vi "4461 - Create AO waveforms.vi"(8 "error in (no error)":errorcluster, 10 "reset phase":bool, 11 "Lockin.DAQ":refnum<class "Lockin.DAQ.lvclass">) -> (0 "error out":errorcluster, 2 "AO Array":waveform(dbl)[](array[waveform]), 3 "Lockin.DAQ":refnum<class "Lockin.DAQ.lvclass">)   [LabVIEW 2016, in "Lockin.DAQ.lvclass"]
uses:
  Lockin.DAQ.lvclass
  Typedefs/AO-cluster.ctl
  Instrument.Lockinl.UI/Typedefs/AO Channel--Cluster.ctl
  Typedefs/Function-enum.ctl
  Lockin.DAQ.lvclass/Lockin.DAQ.ctl
  <vilib>/measure/NI_MABase.lvlib
  Typedefs/Sampling.ctl
  Instrument.Lockinl.UI/Instrument.Lockin.UI.lvclass
panel:
  in  "Channels: AO":T1 {"Phase" format="%.3g"; "Frequency" min=0.0001 max=10000.0 format="%.3g"; "Offset" format="%.3p"; "Amplitude" min=0.0 max=10.0 format="%.3p"}
  in  "Update Graph?":bool
  out "Waveform Chart":dbl[][](graph)
  out "Waveform Graph":waveform(dbl)[](graph)
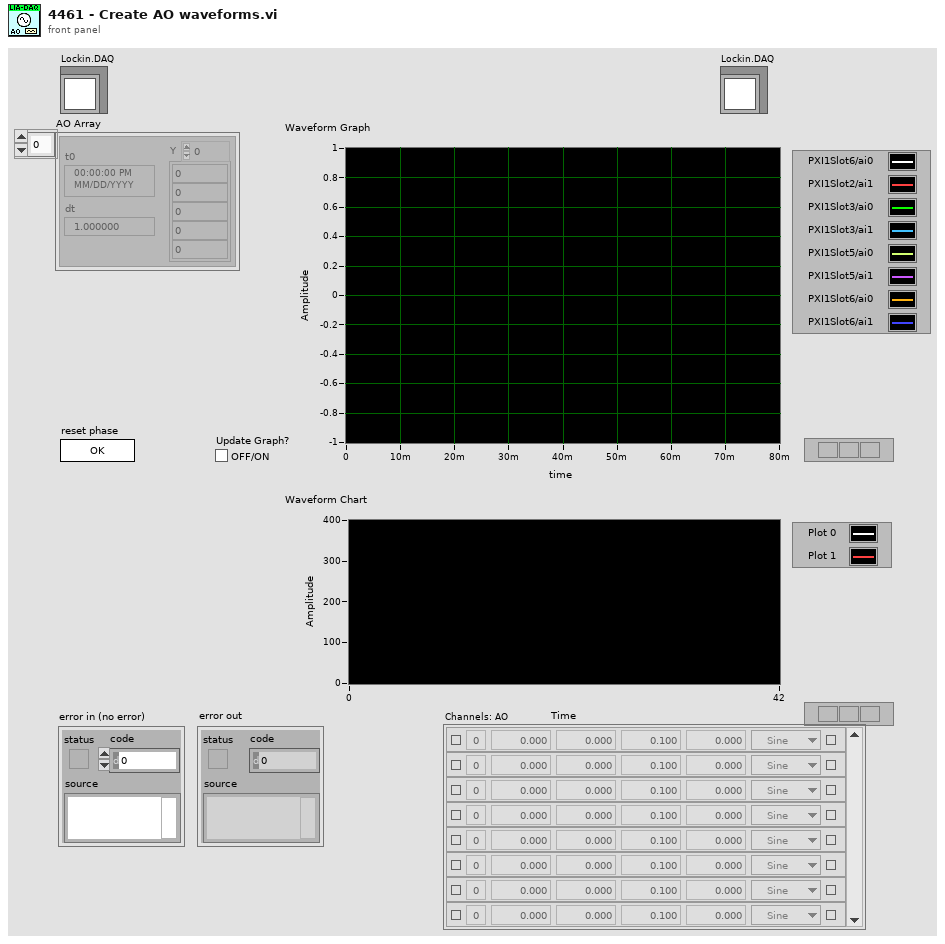
[diagram p1: front panel]
types:
  T1 = typedef "Lockin.DAQ.lvclass/AO-cluster.ctl" = T2[]
  T2 = typedef "Instrument.Lockin.UI.lvclass/AO Channel--Cluster.ctl" = cluster{"Enable?":bool, "Channel":i32, "Amplitude":dbl, "Offset":dbl, "Frequency":dbl, "Phase":dbl, "Function":T3, "Sweeping?":bool}
  T3 = typedef "Lockin.DAQ.lvclass/Function-enum.ctl" = enum16{"Sine", "Triangle", "Square"}
  T4 = typedef "Lockin.DAQ.lvclass/Sampling.ctl" = cluster{"Fs":dbl, "#s":i32}
  T5 = enum16{"Sine Wave", "Triangle Wave", "Square Wave", "Sawtooth Wave"}
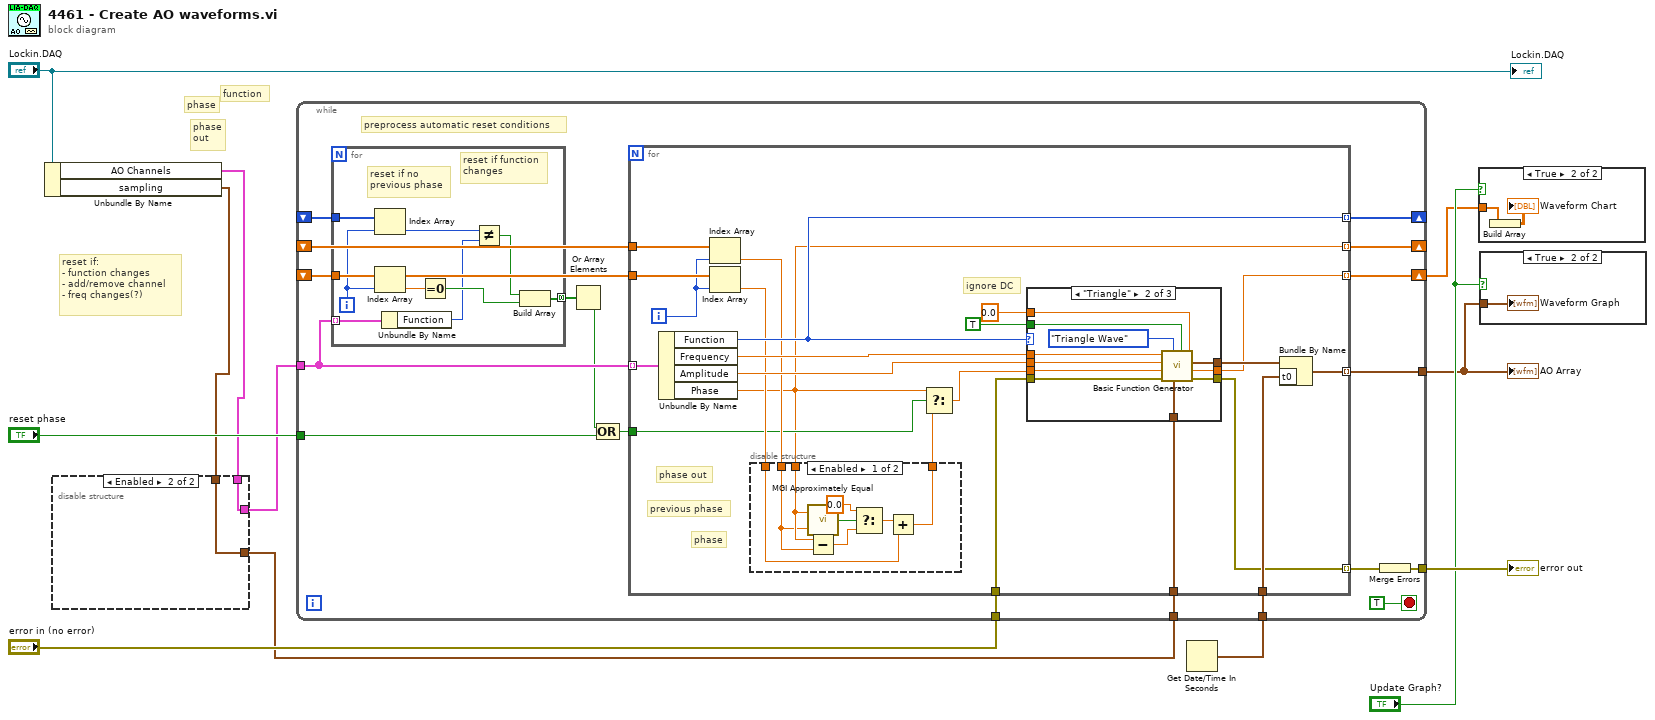
[diagram p0: block diagram]
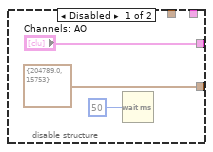
[diagram p2: hidden frame]
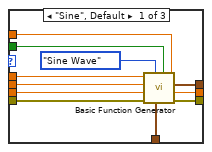
[diagram p4: hidden frame]
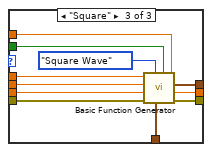
[diagram p5: hidden frame]
diagram:
  # "phase"
  # "function"
  # "phase\nout"
  # "reset if:\n- function changes\n- add/remove channel\n- freq changes(?)"
  n1 = Unbundle By Name("Lockin.DAQ") -> ("AO Channels"=w2:T1, "sampling"=w1:T4)
  n2 = disable-structure shown="Enabled" {
    disable-tunnel: [T4 {"Fs"=204789.0, "#s"=15753} ("Configuration.DAQ.sampling") w16] -> w4
    disable-tunnel: ["Channels: AO" w17] -> w3
    disable-tunnel: w2 -> [_ w17]
    disable-tunnel: w1 -> [_ w16]
    frame Disabled {
      n3 = Wait (ms)(milliseconds to wait=u32 50) -> ()  [unwired: 1 out]
    }
    frame Enabled {
    }
  }
  n4 = Get Date/Time In Seconds() -> (seconds since 1Jan1904=w11:timestamp)
  n5 = while {
    tunnel: w4 -> [w35]
    tunnel: [w34] -> w6
    shift-right: [w32] -> w5
    shift-left: _ -> [w20]
    tunnel: w11 -> [w31]
    tunnel: "reset phase" -> [w24]
    tunnel: "error in (no error)" -> [w30]
    tunnel: [w28] -> w10
    tunnel: w3 -> [w27]
    shift-right: [w22] -> _
    shift-left: _ -> [w21]
    shift-right: [w19] -> _
    shift-left: _ -> [w18]
    stop <- TRUE stop-if-true
    # "preprocess automatic reset conditions"
    n6 = for {
      tunnel: w27 -> [w37] mode=indexing
      tunnel: w20 -> [w44]
      tunnel: w21 -> [w43]
      tunnel: [w38] -> w26 mode=concatenating
      i -> [w45]
      # "reset if function\nchanges"
      # "reset if no\nprevious phase"
      n7 = Index Array(array=w43, index=w45) -> (element=w41:T3)
      n8 = Index Array(array=w44, index=w45) -> (element=w42:dbl)
      n9 = Unbundle By Name(w37) -> ("Function"=w36:T3)
      n10 = Equal To 0?(x=w42) -> (x = 0?=w39:bool)
      n11 = Not Equal?(x=w41, y=w36) -> (x != y?=w40:bool)
      n12 = Build Array(w40, w39) -> (w38:bool[])
    }
    n13 = Or Array Elements(Boolean array=w26) -> (logical OR=w25:bool)
    n14 = Compound Arithmetic op=OR(w25, w24) -> (w23:bool)
    n15 = for {
      tunnel: [w64] -> w34 mode=indexing
      tunnel: w35 -> [w61]
      tunnel: [w62] -> w32 mode=indexing
      tunnel: w31 -> [w66]
      tunnel: w30 -> [w59]
      tunnel: [w63] -> w29 mode=indexing
      tunnel: w27 -> [w58] mode=indexing
      tunnel: w23 -> [w47]
      tunnel: [w55] -> w22 mode=indexing
      tunnel: w20 -> [w54]
      tunnel: [w46] -> w19 mode=indexing
      tunnel: w18 -> [w50]
      i -> [w53]
      # "previous phase"
      # "phase"
      # "phase out"
      # "ignore DC"
      n16 = Unbundle By Name(w58) -> ("Function"=w55:T3, "Frequency"=w56:dbl, "Amplitude"=w57:dbl, "Phase"=w46:dbl)
      n17 = Index Array(array=w50, index=w53) -> (element=w51:dbl)
      n18 = Index Array(array=w54, index=w53) -> (element=w52:dbl)
      n19 = disable-structure shown="Enabled" {
        disable-tunnel: w46 -> [w74 _]
        disable-tunnel: w51 -> [w73 _]
        disable-tunnel: w52 -> [w68 w76]
        disable-tunnel: [w71 w76] -> w49
        frame Enabled {
          n20 = call <userlib>:"MGI Approximately Equal.vi"("Numeric 2"=w73, "Numeric 1"=w74) -> ("approx = ?"=w72:bool)
          n21 = Subtract(x=w74, y=w73) -> (x-y=w70:dbl)
          n22 = Select(t=0.0, s=w72, f=w70) -> (s? t:f=w69:dbl)
          n23 = Add(x=w69, y=w68) -> (x+y=w71:dbl)
        }
        frame Disabled {
        }
      }
      n24 = Select(t=w46, s=w47, f=w49) -> (s? t:f=w48:dbl)
      n25 = case shown="\"Triangle\"" w55 {
        tunnel: w56 -> [w87 w98 w109]
        tunnel: 0.0 ("AO DC") -> [w86 w97 w108]
        tunnel: [w85 w96 w107] -> w67
        tunnel: TRUE ("reset signal") -> [w77 w88 w99]
        tunnel: w59 -> [w84 w95 w106]
        tunnel: [w83 w94 w105] -> w63
        tunnel: [w82 w93 w104] -> w62
        tunnel: w57 -> [w81 w92 w103]
        tunnel: w48 -> [w80 w91 w102]
        tunnel: w61 -> [w79 w90 w101]
        frame "Sine", Default {
          n26 = call <vilib>:"Basic Function Generator.vi"("offset"=w86, "reset signal"=w77, "sampling info"=w79, "signal type"=T5."Sine Wave", "error in (no error)"=w84, "phase"=w80, "amplitude"=w81, "frequency"=w87) -> ("error out"=w83:errorcluster, "phase out"=w82:dbl, "signal out"=w85:waveform(dbl))  [unwired: 1 in]
        }
        frame "Triangle" {
          n27 = call <vilib>:"Basic Function Generator.vi"("offset"=w97, "reset signal"=w88, "sampling info"=w90, "signal type"=T5."Triangle Wave", "error in (no error)"=w95, "phase"=w91, "amplitude"=w92, "frequency"=w98) -> ("error out"=w94:errorcluster, "phase out"=w93:dbl, "signal out"=w96:waveform(dbl))  [unwired: 1 in]
        }
        frame "Square" {
          n28 = call <vilib>:"Basic Function Generator.vi"("offset"=w108, "reset signal"=w99, "sampling info"=w101, "signal type"=T5."Square Wave", "error in (no error)"=w106, "phase"=w102, "amplitude"=w103, "frequency"=w109) -> ("error out"=w105:errorcluster, "phase out"=w104:dbl, "signal out"=w107:waveform(dbl))  [unwired: 1 in]
        }
      }
      n29 = Bundle By Name(cluster=w67, "t0"=w66) -> (w64:waveform(dbl))
    }
    n30 = Merge Errors(w29) -> (w28:errorcluster)
  }
  "AO Array" <- w6
  "error out" <- w10
  n31 = case shown="True" "Update Graph?" {
    tunnel: w5 -> [_ w111]
    frame False {
    }
    frame True {
      n32 = Build Array(w111) -> (→"Waveform Chart":dbl[][])
    }
  }
  n33 = case shown="True" "Update Graph?" {
    tunnel: w6 -> [_ w112]
    frame False {
    }
    frame True {
      "Waveform Graph" <- w112
    }
  }
  "Lockin.DAQ" <- "Lockin.DAQ"
